vi "1553_RT_GetMessages_Test.vi"() -> ()   [LabVIEW 2020]
panel:
  in  "EmptyArray":bool
  out "Message box":string[][](table)
  out "RT Msg Data (In)":u16[](array[numeric]) format="%04x"
  in  "Blknum":i32=1 min=0 max=199
  in  "Stop":bool
  in  "Transmit/Receive":i32(ring) items=["Receive", "Transmit"]
  in  "RT Subaddress":i32=1 min=0 max=31
  in  "RT Num":i32=1 min=0 max=31
  out "Mode.Get":i32(ring) items=["RT"=2, "BC/CONCURRENT RT"=4, "MONITOR - BLOCK"=8, "MONITOR - LOOKUP"=32, "LL 0018"=68]
  out "FW Revision":i32
  out "Module Id":i32
  out "Board Status Flags":string[](array[string])
  in  "Mode":i32(ring)=2 items=["RT"=2, "BC/CONCURRENT RT"=4, "MONITOR - BLOCK"=8, "MONITOR - LOOKUP"=32, "LL 0018"=68]
  out "Card Initialized":bool=TRUE
  in  "Module":u16=1
  in  "Device":u16 max=255 step=1
  out "error out":errorcluster
  in  "error in":errorcluster
  # "INITIALIZE"
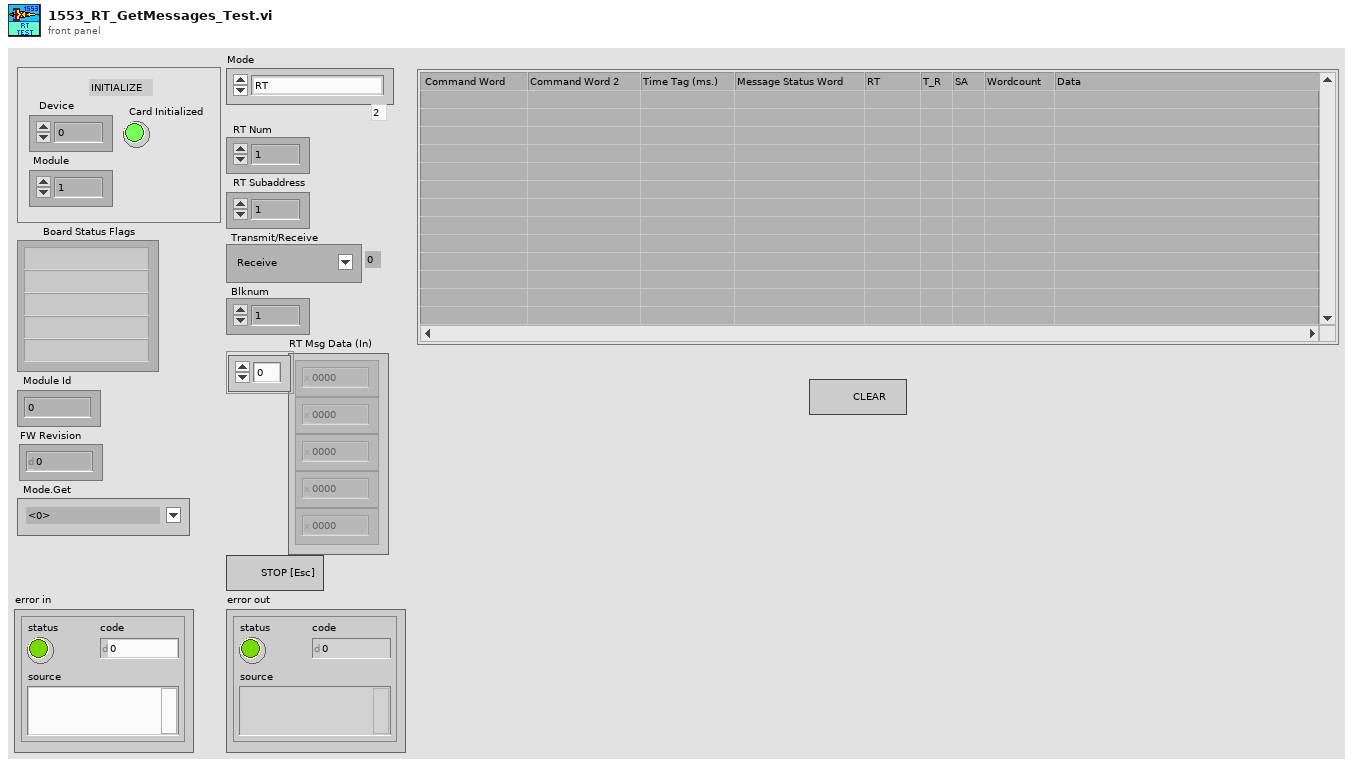
[diagram p1: front panel]
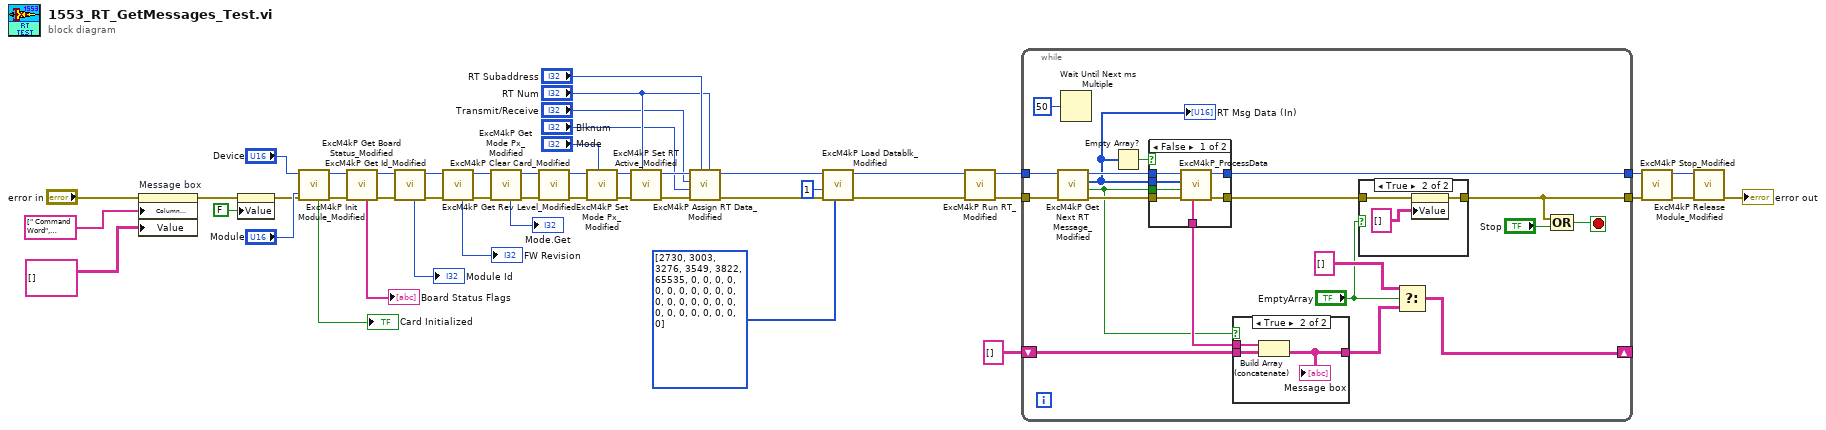
[diagram p0: block diagram]
diagram:
  n1 = property on="Message box" class="Tbl (strict)"(error in="error in", "Column Headers[]"=string[] [" Command Word", "Command Word 2", "Time Tag (ms.)", "Message Status Word", "RT", "T_R", "SA", "Wordcount", "Data", ""] ("Column Header Strings[]"), "Value"=string[][] [] ("Message box")) -> (error out=w10:errorcluster)  [unwired: 1 in, 1 out]
  n2 = property on="Card Initialized" class="Bool (strict)"(error in=w10, "Value"=FALSE ("Card Initialized")) -> (error out=w45:errorcluster)  [unwired: 1 in, 1 out]
  n3 = call "ExcM4kP Init Module_Modified.vi"("Module"="Module", "error in (no error)"=w45, "Device"="Device") -> ("error out"=w39:errorcluster, "Handle"=w40:u32, "Card Initialized"=→"Card Initialized":bool)  [unwired: 6 in]
  n4 = call "ExcM4kP Get Board Status_Modified.vi"("error in (no error)"=w39, "Handle.In"=w40) -> ("error out"=w36:errorcluster, "Handle.DUP"=w37:u32, "Board Status Flags"=→"Board Status Flags":string[])  [unwired: 6 in, 1 out]
  n5 = call "ExcM4kP Get Id_Modified.vi"("error in (no error)"=w36, "Handle.In"=w37) -> ("error out"=w33:errorcluster, "Handle.DUP"=w34:u32, "Module Id"=→"Module Id":i32)  [unwired: 7 in]
  n6 = call "ExcM4kP Get Rev Level_Modified.vi"("error in (no error)"=w33, "Handle.In"=w34) -> ("error out"=w31:errorcluster, "Handle.DUP"=w30:u32, "Board.FW.Revision"=→"FW Revision":i32)  [unwired: 7 in]
  n7 = call "ExcM4kP Get Mode Px_Modified.vi"("error in (no error)"=w31, "Handle.In"=w30) -> ("error out"=w25:errorcluster, "Handle.DUP"=w27:u32, "Mode"=→"Mode.Get":i32)  [unwired: 7 in]
  n8 = call "ExcM4kP Clear Card_Modified.vi"("error in (no error)"=w25, "Handle.In"=w27) -> ("error out"=w24:errorcluster, "Handle.DUP"=w26:u32)  [unwired: 8 in]
  n9 = call "ExcM4kP Set Mode Px_Modified.vi"("Mode"="Mode", "error in (no error)"=w24, "Handle.In"=w26) -> ("error out"=w23:errorcluster, "Handle.DUP"=w22:u32)  [unwired: 7 in]
  n10 = call "ExcM4kP Set RT Active_Modified.vi"("RT Num"="RT Num", "error in (no error)"=w23, "Handle.In"=w22) -> ("error out"=w21:errorcluster, "Handle.DUP"=w20:u32)  [unwired: 7 in]
  n11 = call "ExcM4kP Assign RT Data_Modified.vi"("RT Address"="RT Num", "RT Subaddress"="RT Subaddress", "error in (no error)"=w21, "Blknum"="Blknum", "Transmit/Receive"="Transmit/Receive", "Handle.In"=w20) -> ("error out"=w7:errorcluster, "Handle.DUP"=w5:u32)  [unwired: 4 in]
  n12 = call "ExcM4kP Load Datablk_Modified.vi"("Data"=u16[] [2730, 3003, 3276, 3549, 3822, 65535, 0, 0, 0, 0, 0, 0, 0, 0, 0, 0, 0, 0, 0, 0, 0, 0, 0, 0, 0, 0, 0, 0, 0, 0, 0, 0], "error in (no error)"=w7, "Blknum"=1, "Handle.In"=w5) -> ("error out"=w6:errorcluster, "Handle.DUP"=w4:u32)  [unwired: 6 in]
  n13 = call "ExcM4kP Run RT_Modified.vi"("error in (no error)"=w6, "Handle.In"=w4) -> ("error out"=w16:errorcluster, "Handle.DUP"=w14:u32)  [unwired: 8 in]
  n14 = while {
    tunnel: w14 -> [w66]
    tunnel: [w57] -> w13
    tunnel: w16 -> [w67]
    tunnel: [w52] -> w15
    shift-right: [w54] -> _
    shift-left: string[][] [] -> [w60]
    stop <- w64 stop-if-true
    n15 = call "ExcM4kP Get Next RT Message_Modified.vi"("error in (no error)"=w67, "Handle.In"=w66) -> ("error out"=w61:errorcluster, "Msg Returned Flag"=w58:bool, "RT Msg Data"=w49:u16[], "Handle.DUP"=w62:u32)  [unwired: 5 in, 1 out]
    "RT Msg Data (In)" <- w49
    n16 = Wait Until Next ms Multiple(millisecond multiple=u32 50) -> ()  [unwired: 1 out]
    n17 = Empty Array?(array=w49) -> (empty?=w50:bool)
    n18 = case shown="False" w50 {
      tunnel: w62 -> [w74 w76]
      tunnel: w61 -> [w73 w75]
      tunnel: w49 -> [w72 _]
      tunnel: [w71 _] -> w59
      tunnel: w58 -> [w70 _]
      tunnel: [w69 w76] -> w57
      tunnel: [w68 w75] -> w53
      frame False {
        n19 = call "ExcM4kP_ProcessData.vi"("error in (no error)"=w73, "Msg Returned Flag"=w70, "Data"=w72, "Handle.In"=w74) -> ("error out"=w68:errorcluster, "Handle.DUP"=w69:u32, "Message.Array"=w71:string[])  [unwired: 3 in, 2 out]
      }
      frame True {
      }
    }
    n20 = case shown="True" w58 {
      tunnel: w60 -> [w81 w84]
      tunnel: w59 -> [_ w83]
      tunnel: [w81 w82] -> w55
      frame False {
      }
      frame True {
        n21 = Build Array (concatenate)(w83, w84) -> (w82:string[][])
        "Message box" <- w82
      }
    }
    n22 = case shown="True" "EmptyArray" {
      tunnel: w53 -> [w77 w80]
      tunnel: [w77 w79] -> w52
      frame False {
      }
      frame True {
        n23 = property on="Message box" class="Tbl (strict)"(error in=w80, "Value"=string[][] [] ("t")) -> (error out=w79:errorcluster)  [unwired: 1 in, 1 out]
      }
    }
    n24 = Select(t=string[][] [], s="EmptyArray", f=w55) -> (s? t:f=w54:string[][])
    n25 = Compound Arithmetic op=OR(w52, "Stop") -> (w64:bool)
  }
  n26 = call "ExcM4kP Stop_Modified.vi"("error in (no error)"=w15, "Handle.In"=w13) -> ("error out"=w42:errorcluster, "Handle.DUP"=w41:u32)  [unwired: 8 in]
  n27 = call "ExcM4kP Release Module_Modified.vi"("error in (no error)"=w42, "Handle.In"=w41) -> ("error out"=→"error out":errorcluster)  [unwired: 9 in]
